vi "Get number of summed images value in CameraParameterSetup.vi"(0 "CameraParametersSetup":T1[](array[typedef])) -> (4 "CameraParametersSetup (dup)":T1[](array[typedef]), 6 "nb_summed_images":i32)   [LabVIEW 2020]
uses:
  CameraParametersSetup.ctl
  CameraParameters_Type.ctl
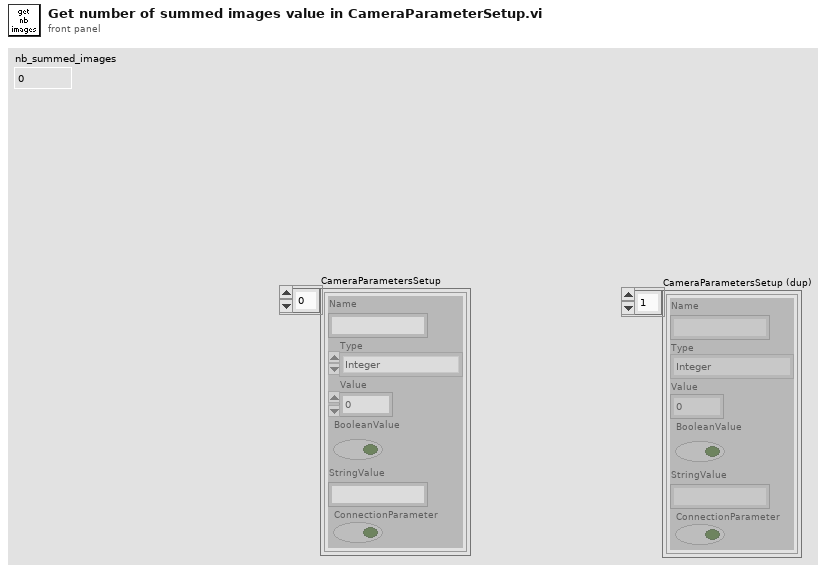
[diagram p1: front panel]
types:
  T1 = typedef "CameraParametersSetup.ctl" = cluster{"Name":string, "Type":T2, "Value":dbl, "BooleanValue":bool, "StringValue":string, "ConnectionParameter":bool}
  T2 = typedef "CameraParameters_Type.ctl" = enum16{"Integer", "Real", "String", "Boolean"}
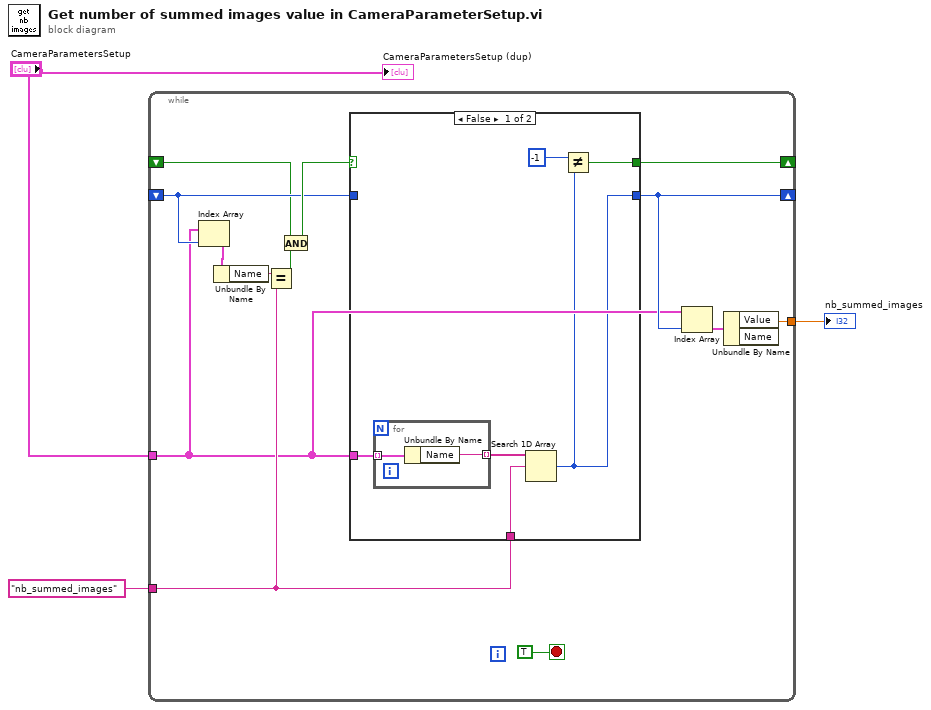
[diagram p0: block diagram]
diagram:
  n1 = while {
    tunnel: "CameraParametersSetup" -> [w7]
    shift-right: [w16] -> _
    shift-left: _ -> [w8]
    tunnel: [w14] -> w3
    shift-right: [w5] -> _
    shift-left: _ -> [w6]
    tunnel: "nb_summed_images" -> [w9]
    stop <- TRUE stop-if-true
    n2 = Index Array(array=w7, index=w8) -> (element=w13:T1)
    n3 = Unbundle By Name(w13) -> ("Name"=w12:string)
    n4 = Equal?(x=w12, y=w9) -> (x = y?=w11:bool)
    n5 = And(x=w6, y=w11) -> (x .and. y?=w10:bool)
    n6 = case shown="False" w10 {
      selector: w10 -> [_ w25]
      tunnel: w7 -> [w22 _]
      tunnel: [w19 w26] -> w16
      tunnel: w8 -> [_ w26]
      tunnel: [w18 w25] -> w5
      tunnel: w9 -> [w17 _]
      frame False {
        n7 = for {
          tunnel: w22 -> [w24] mode=indexing
          tunnel: [w23] -> w21 mode=indexing
          n8 = Unbundle By Name(w24) -> ("Name"=w23:string)
        }
        n9 = Search 1D Array(1D array=w21, element=w17) -> (index of element=w19:i32)  [unwired: 1 in]
        n10 = Not Equal?(x=-1, y=w19) -> (x != y?=w18:bool)
      }
      frame True {
      }
    }
    n11 = Index Array(array=w7, index=w16) -> (element=w15:T1)
    n12 = Unbundle By Name(w15) -> ("Value"=w14:dbl)  [unwired: 1 out]
  }
  "nb_summed_images" <- w3
  "CameraParametersSetup (dup)" <- "CameraParametersSetup"
